vi "SRV_Sensor Config Control Attributes.vi"(8 "error in (no error)":errorcluster, 10 "Sensors Config GUI":T9={"Sensor Config Index 0"={"Name"="Button xx", "A/D"=enum."Analog", "I2C Address"=0, "Register"=0, "Channel"=0, "Digital Mask"=0, "Units"="", "Sampling Mode"=enum."Polled", "Sample Period (ms)"=1000, "Formula"="", "Sensor View Config"={"Sensor Name"=enum."Gauge 01", "Minimum"=0.0, "Maximum"=10.0}, "Active"=FALSE, "PicoC Shared Var Type"=enum."Integer", "Index"=0, "Stream Multiple?"=FALSE, "Index End"=255, "Bytes"=enum."1 Byte", "Source Sensor Name"="", "Repeat Start"=FALSE, "Integer Word Type"=enum."Unsigned", "Byte Swap"=FALSE}, "Sensor Config Index 1"={"Name"="Button xx", "A/D"=enum."Analog", "I2C Address"=0, "Register"=0, "Channel"=0, "Digital Mask"=0, "Units"="", "Sampling Mode"=enum."Polled", "Sample Period (ms)"=1000, "Formula"="", "Sensor View Config"={"Sensor Name"=enum."Gauge 01", "Minimum"=0.0, "Maximum"=10.0}, "Active"=FALSE, "PicoC Shared Var Type"=enum."Integer", "Index"=0, "Stream Multiple?"=FALSE, "Index End"=255, "Bytes"=enum."1 Byte", "Source Sensor Name"="", "Repeat Start"=FALSE, "Integer Word Type"=enum."Unsigned", "Byte Swap"=FALSE}, "Sensor Config Index 2"={"Name"="Button xx", "A/D"=enum."Analog", "I2C Address"=0, "Register"=0, "Channel"=0, "Digital Mask"=0, "Units"="", "Sampling Mode"=enum."Polled", "Sample Period (ms)"=1000, "Formula"="", "Sensor View Config"={"Sensor Name"=enum."Gauge 01", "Minimum"=0.0, "Maximum"=10.0}, "Active"=FALSE, "PicoC Shared Var Type"=enum."Integer", "Index"=0, "Stream Multiple?"=FALSE, "Index End"=255, "Bytes"=enum."1 Byte", "Source Sensor Name"="", "Repeat Start"=FALSE, "Integer Word Type"=enum."Unsigned", "Byte Swap"=FALSE}} {"Sensor Config Index 2"."Register" format="%.0x"; "Sensor Config Index 2"."I2C Address" format="%.0x"; "Sensor Config Index 2"."Sample Period (ms)" min=10 max=60000 step=1; "Sensor Config Index 2"."Digital Mask" format="%.0x"; "Sensor Config Index 2"."Channel" format="%.0x"; "Sensor Config Index 1"."Register" format="%.0x"; "Sensor Config Index 1"."I2C Address" format="%.0x"; "Sensor Config Index 1"."Sample Period (ms)" min=10 max=60000 step=1; "Sensor Config Index 1"."Digital Mask" format="%.0x"; "Sensor Config Index 1"."Channel" format="%.0x"; "Sensor Config Index 0"."Register" format="%.0x"; "Sensor Config Index 0"."I2C Address" format="%.0x"; "Sensor Config Index 0"."Sample Period (ms)" min=10 max=60000 step=1; "Sensor Config Index 0"."Digital Mask" format="%.0x"; "Sensor Config Index 0"."Channel" format="%.0x"}, 11 "Sensor Config Control refs":T10) -> (0 "error out":errorcluster)   [LabVIEW 2014]
uses:
  SRV_Sensor Config Control refs.ctl
  SRV_Sensor Config Cluster.ctl
  SRV_Sensor Analog-Digital.ctl
  SRV_Sensor Sampling Mode.ctl
  SRV_Sensor View Config Cluster.ctl
  SRV_Sensors Names.ctl
  SRV_Sensor PicoC Shared Var Type.ctl
  SRV_Sensor Number of Bytes.ctl
  SRV_Sensor Integer Word Type.ctl
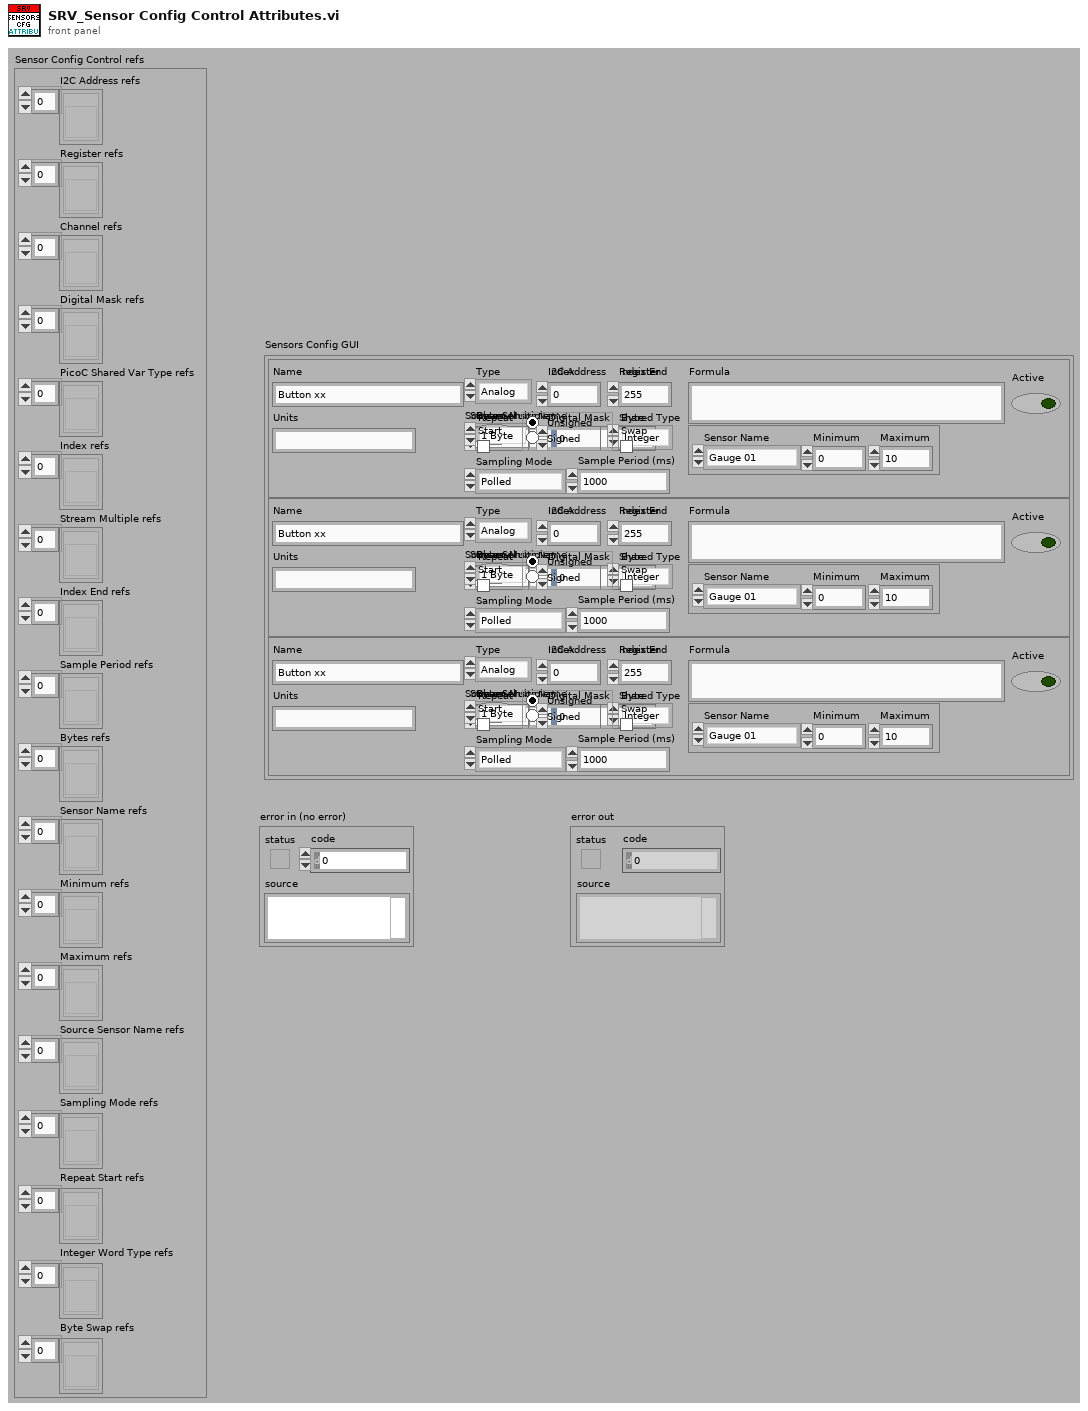
[diagram p1: front panel]
types:
  T1 = typedef "SRV_Sensor Config Cluster.ctl" = cluster{"Name":string, "A/D":T2, "I2C Address":u8, "Register":u8, "Channel":u8, "Digital Mask":u16, "Units":string, "Sampling Mode":T3, "Sample Period (ms)":u32, "Formula":string, "Sensor View Config":T4, "Active":bool, "PicoC Shared Var Type":T6, "Index":u8, "Stream Multiple?":bool, "Index End":u8, "Bytes":T7, "Source Sensor Name":string, "Repeat Start":bool, "Integer Word Type":T8, "Byte Swap":bool}
  T2 = typedef "SRV_Sensor Analog-Digital.ctl" = enum16{"Digital", "Analog", "PicoC Shared", "Calculated"}
  T3 = typedef "SRV_Sensor Sampling Mode.ctl" = enum16{"Polled", "Streaming"}
  T4 = typedef "SRV_Sensor View Config Cluster.ctl" = cluster{"Sensor Name":T5, "Minimum":dbl, "Maximum":dbl}
  T5 = typedef "SRV_Sensors Names.ctl" = enum16{"Gauge 01", "Gauge 02", "Gauge 03", "Gauge 04", "Meter 01", "Meter 02", "Meter 03", "Meter 04", "Numeric 01", "Numeric 02", "Numeric 03", "Numeric 04", "Numeric 05", "Numeric 06", "Numeric 07", "Numeric 08", "Boolean 01", "Boolean 02", "Boolean 03", "Boolean 04", "Boolean 05", "Boolean 06", "Boolean 07", "Boolean 08", "Boolean 09", "Boolean 10", "Boolean 11", "Boolean 12", "Boolean 13", "Boolean 14", "Boolean 15", "Boolean 16", "Boolean 17", "Boolean 18", "Boolean 19", "Boolean 20", "Boolean 21", "Boolean 22", "Boolean 23", "Boolean 24", "Boolean 25", "Boolean 26", "Boolean 27", "Boolean 28", "Boolean 29", "Boolean 30", "Boolean 31", "Boolean 32"}
  T6 = typedef "SRV_Sensor PicoC Shared Var Type.ctl" = enum16{"String", "Integer", "Float"}
  T7 = typedef "SRV_Sensor Number of Bytes.ctl" = enum16{"1 Byte", "2 Bytes"}
  T8 = typedef "SRV_Sensor Integer Word Type.ctl" = enum32{"Unsigned", "Signed"}
  T9 = cluster{"Sensor Config Index 0":T1, "Sensor Config Index 1":T1, "Sensor Config Index 2":T1}
  T10 = typedef "SRV_Sensor Config Control refs.ctl" = cluster{"I2C Address refs":refnum<vi>[], "Register refs":refnum<vi>[], "Channel refs":refnum<vi>[], "Digital Mask refs":refnum<vi>[], "PicoC Shared Var Type refs":refnum<vi>[], "Index refs":refnum<vi>[], "Stream Multiple refs":refnum<vi>[], "Index End refs":refnum<vi>[], "Sample Period refs":refnum<vi>[], "Bytes refs":refnum<vi>[], "Sensor Name refs":refnum<vi>[], "Minimum refs":refnum<vi>[], "Maximum refs":refnum<vi>[], "Source Sensor Name refs":refnum<vi>[], "Sampling Mode refs":refnum<vi>[], "Repeat Start refs":refnum<vi>[], "Integer Word Type refs":refnum<vi>[], "Byte Swap refs":refnum<vi>[]}
  T11 = enum8{"Enabled", "Disabled", "Disabled and Grayed Out"}
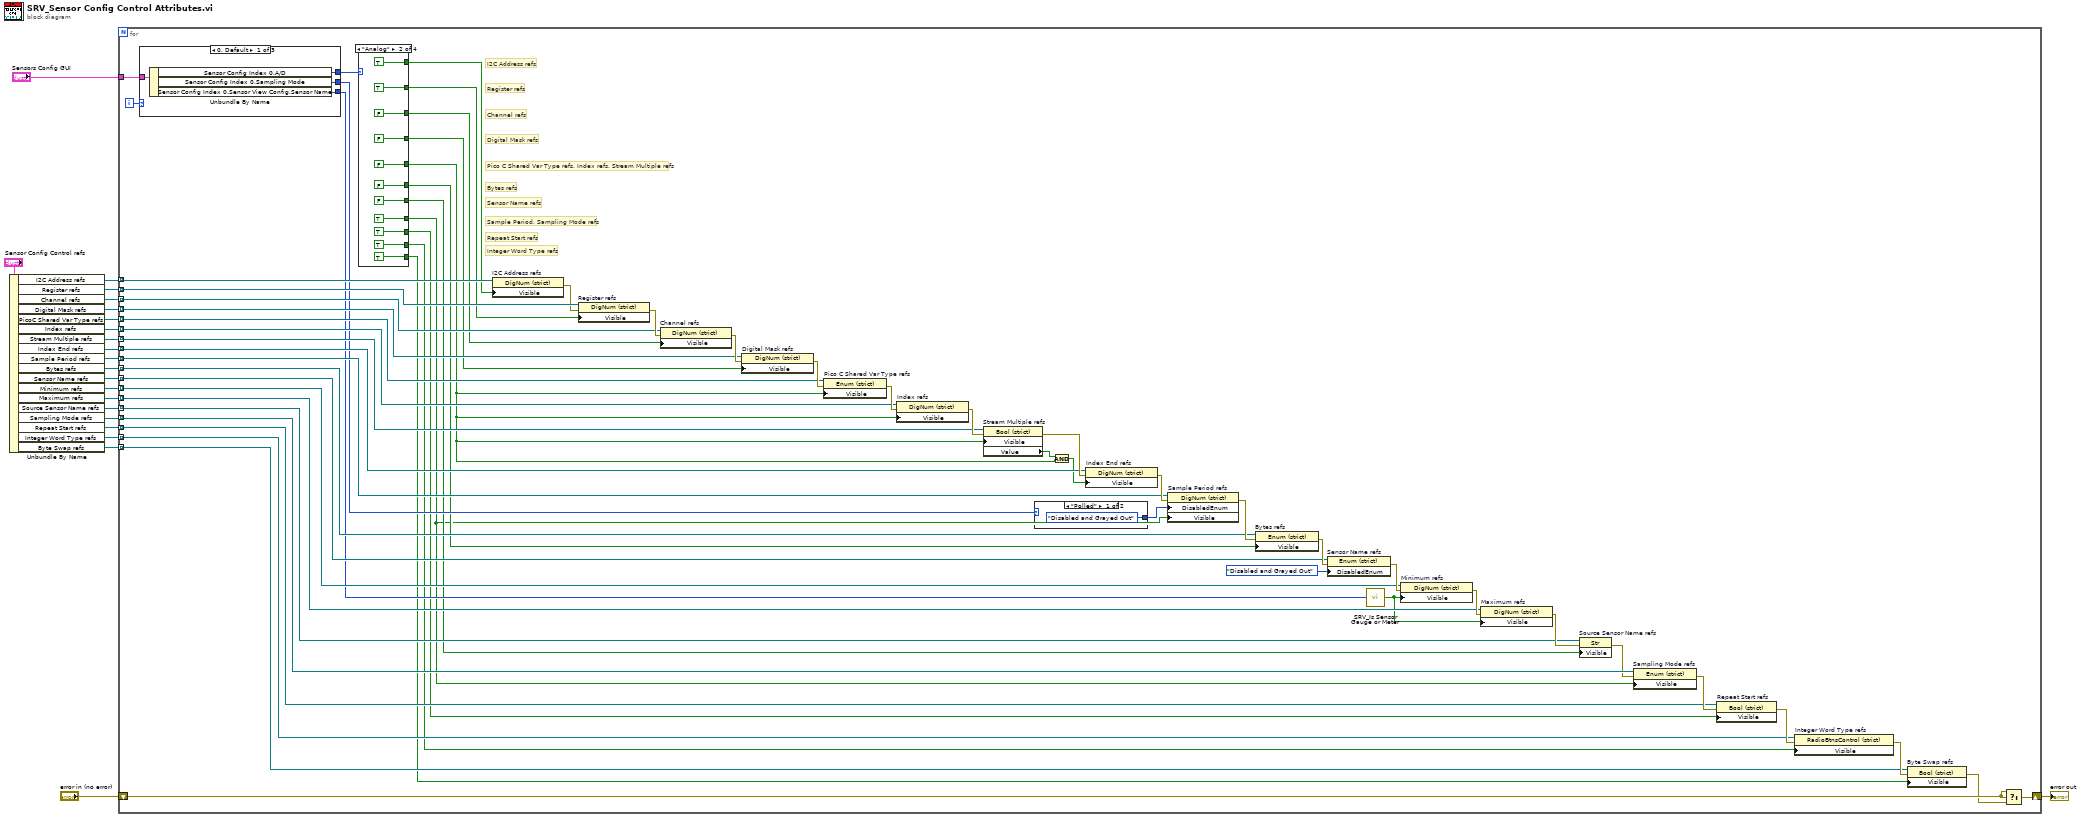
[diagram p0: block diagram]
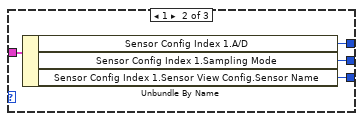
[diagram p2: hidden frame]
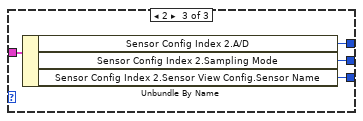
[diagram p3: hidden frame]
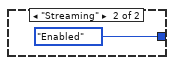
[diagram p4: hidden frame]
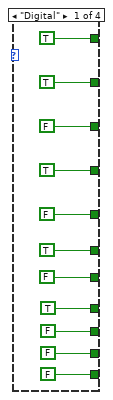
[diagram p5: hidden frame]
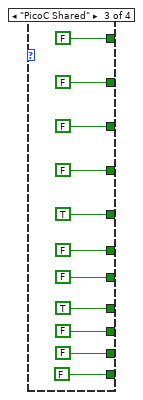
[diagram p6: hidden frame]
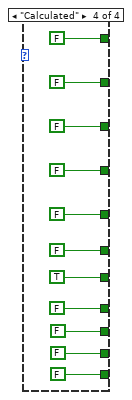
[diagram p7: hidden frame]
diagram:
  n1 = Unbundle By Name("Sensor Config Control refs") -> ("I2C Address refs"=w21:refnum<vi>[], "Register refs"=w20:refnum<vi>[], "Channel refs"=w19:refnum<vi>[], "Digital Mask refs"=w18:refnum<vi>[], "PicoC Shared Var Type refs"=w17:refnum<vi>[], "Index refs"=w16:refnum<vi>[], "Stream Multiple refs"=w15:refnum<vi>[], "Index End refs"=w14:refnum<vi>[], "Sample Period refs"=w11:refnum<vi>[], "Bytes refs"=w9:refnum<vi>[], "Sensor Name refs"=w8:refnum<vi>[], "Minimum refs"=w7:refnum<vi>[], "Maximum refs"=w6:refnum<vi>[], "Source Sensor Name refs"=w5:refnum<vi>[], "Sampling Mode refs"=w4:refnum<vi>[], "Repeat Start refs"=w3:refnum<vi>[], "Integer Word Type refs"=w2:refnum<vi>[], "Byte Swap refs"=w1:refnum<vi>[])
  n2 = for {
    tunnel: "Sensors Config GUI" -> [w80]
    tunnel: w21 -> [w79] mode=indexing
    tunnel: w20 -> [w78] mode=indexing
    tunnel: w19 -> [w73] mode=indexing
    tunnel: w18 -> [w70] mode=indexing
    tunnel: w17 -> [w67] mode=indexing
    tunnel: w16 -> [w65] mode=indexing
    tunnel: w15 -> [w63] mode=indexing
    tunnel: w14 -> [w59] mode=indexing
    shift-right: [w56] -> w12
    shift-left: "error in (no error)" -> [w57]
    tunnel: w11 -> [w54] mode=indexing
    tunnel: w9 -> [w49] mode=indexing
    tunnel: w8 -> [w44] mode=indexing
    tunnel: w7 -> [w43] mode=indexing
    tunnel: w6 -> [w42] mode=indexing
    tunnel: w5 -> [w37] mode=indexing
    tunnel: w4 -> [w35] mode=indexing
    tunnel: w3 -> [w30] mode=indexing
    tunnel: w2 -> [w29] mode=indexing
    tunnel: w1 -> [w24] mode=indexing
    i -> [w51]
    # "Integer Word Type refs"
    # "Repeat Start refs"
    # "Sample Period, Sampling Mode refs"
    # "Sensor Name refs"
    # "Bytes refs"
    # "Pico C Shared Var Type refs, Index refs, Stream Multiple refs"
    # "Digital Mask refs"
    # "Channel refs"
    # "Register refs"
    # "I2C Address refs"
    n3 = case shown="0, Default" w51 {
      tunnel: [w84 w89 w93] -> w81
      tunnel: w80 -> [w85 w88 w92]
      tunnel: [w83 w87 w91] -> w53
      tunnel: [w82 w86 w90] -> w39
      frame 0, Default {
        n4 = Unbundle By Name(w85) -> ("Sensor Config Index 0.A/D"=w84:T2, "Sensor Config Index 0.Sampling Mode"=w83:T3, "Sensor Config Index 0.Sensor View Config.Sensor Name"=w82:T5)
      }
      frame 1 {
        n5 = Unbundle By Name(w88) -> ("Sensor Config Index 1.A/D"=w89:T2, "Sensor Config Index 1.Sampling Mode"=w87:T3, "Sensor Config Index 1.Sensor View Config.Sensor Name"=w86:T5)
      }
      frame 2 {
        n6 = Unbundle By Name(w92) -> ("Sensor Config Index 2.A/D"=w93:T2, "Sensor Config Index 2.Sampling Mode"=w91:T3, "Sensor Config Index 2.Sensor View Config.Sensor Name"=w90:T5)
      }
    }
    n7 = case shown="\"Analog\"" w81 {
      tunnel: [TRUE ("Visible") TRUE ("Visible") FALSE ("Visible") FALSE ("Visible")] -> w76
      tunnel: [TRUE ("Visible") TRUE ("Visible") FALSE ("Visible") FALSE ("Visible")] -> w75
      tunnel: [FALSE ("Visible") FALSE ("Visible") FALSE ("Visible") FALSE ("Visible")] -> w72
      tunnel: [TRUE ("Visible") FALSE ("Visible") FALSE ("Visible") FALSE ("Visible")] -> w69
      tunnel: [FALSE ("Visible") FALSE ("Visible") TRUE ("Visible") FALSE ("Visible")] -> w61
      tunnel: [TRUE ("Visible") FALSE ("Visible") FALSE ("Visible") FALSE ("Visible")] -> w48
      tunnel: [FALSE ("Visible") FALSE ("Visible") FALSE ("Visible") TRUE ("Visible")] -> w36
      tunnel: [TRUE TRUE TRUE FALSE] -> w33
      tunnel: [FALSE TRUE FALSE FALSE] -> w28
      tunnel: [FALSE TRUE FALSE FALSE] -> w27
      tunnel: [FALSE TRUE FALSE FALSE] -> w23
      frame "Digital" {
      }
      frame "Analog" {
      }
      frame "PicoC Shared" {
      }
      frame "Calculated" {
      }
    }
    n8 = property on="I2C Address refs" class="DigNum (strict)"(reference=w79, "Visible"=w76) -> (error out=w77:errorcluster)  [unwired: 1 in, 1 out]
    n9 = property on="Register refs" class="DigNum (strict)"(reference=w78, error in=w77, "Visible"=w75) -> (error out=w74:errorcluster)  [unwired: 1 out]
    n10 = property on="Channel refs" class="DigNum (strict)"(reference=w73, error in=w74, "Visible"=w72) -> (error out=w71:errorcluster)  [unwired: 1 out]
    n11 = property on="Digital Mask refs" class="DigNum (strict)"(reference=w70, error in=w71, "Visible"=w69) -> (error out=w68:errorcluster)  [unwired: 1 out]
    n12 = property on="Pico C Shared Var Type refs" class="Enum (strict)"(reference=w67, error in=w68, "Visible"=w61) -> (error out=w66:errorcluster)  [unwired: 1 out]
    n13 = property on="Index refs" class="DigNum (strict)"(reference=w65, error in=w66, "Visible"=w61) -> (error out=w64:errorcluster)  [unwired: 1 out]
    n14 = property on="Stream Multiple refs" class="Bool (strict)"(reference=w63, error in=w64, "Visible"=w61) -> (error out=w60:errorcluster, "Value"=w62:bool)  [unwired: 1 out]
    n15 = case shown="\"Polled\"" w53 {
      tunnel: [T11."Disabled and Grayed Out" ("Disabled") T11."Enabled" ("Disabled")] -> w52
      frame "Polled" {
      }
      frame "Streaming" {
      }
    }
    n16 = And(x=w62, y=w61) -> (x .and. y?=w58:bool)
    n17 = property on="Index End refs" class="DigNum (strict)"(reference=w59, error in=w60, "Visible"=w58) -> (error out=w55:errorcluster)  [unwired: 1 out]
    n18 = property on="Sample Period refs" class="DigNum (strict)"(reference=w54, error in=w55, "DisabledEnum"=w52, "Visible"=w33) -> (error out=w50:errorcluster)  [unwired: 1 out]
    n19 = property on="Bytes refs" class="Enum (strict)"(reference=w49, error in=w50, "Visible"=w48) -> (error out=w45:errorcluster)  [unwired: 1 out]
    n20 = property on="Sensor Name refs" class="Enum (strict)"(reference=w44, error in=w45, "DisabledEnum"=T11."Disabled and Grayed Out" ("Disabled")) -> (error out=w47:errorcluster)  [unwired: 1 out]
    n21 = call "SRV_Is Sensor Gauge or Meter.vi"("Sensor View Indicator Names"=w39) -> ("Gauge or Meter?"=w40:bool)  [unwired: 14 in]
    n22 = property on="Minimum refs" class="DigNum (strict)"(reference=w43, error in=w47, "Visible"=w40) -> (error out=w46:errorcluster)  [unwired: 1 out]
    n23 = property on="Maximum refs" class="DigNum (strict)"(reference=w42, error in=w46, "Visible"=w40) -> (error out=w38:errorcluster)  [unwired: 1 out]
    n24 = property on="Source Sensor Name refs" class="Str"(reference=w37, error in=w38, "Visible"=w36) -> (error out=w34:errorcluster)  [unwired: 1 out]
    n25 = property on="Sampling Mode refs" class="Enum (strict)"(reference=w35, error in=w34, "Visible"=w33) -> (error out=w31:errorcluster)  [unwired: 1 out]
    n26 = property on="Repeat Start refs" class="Bool (strict)"(reference=w30, error in=w31, "Visible"=w28) -> (error out=w32:errorcluster)  [unwired: 1 out]
    n27 = property on="Integer Word Type refs" class="RadioBtnsControl (strict)"(reference=w29, error in=w32, "Visible"=w27) -> (error out=w26:errorcluster)  [unwired: 1 out]
    n28 = property on="Byte Swap refs" class="Bool (strict)"(reference=w24, error in=w26, "Visible"=w23) -> (error out=w25:errorcluster)  [unwired: 1 out]
    n29 = Select(t=w57, s=w57, f=w25) -> (s? t:f=w56:errorcluster)
  }
  "error out" <- w12
